vi "Deinitialize.vi"(8 "error in":errorcluster, 11 "Channel":u16) -> (0 "error out":errorcluster)   [LabVIEW 2023, in "PCAN API.lvlib"]
doc: "This VI is used to deinitialize a CAN port."
uses:
  PCAN API.lvlib
  PCAN2023/PCAN2023.lvlib
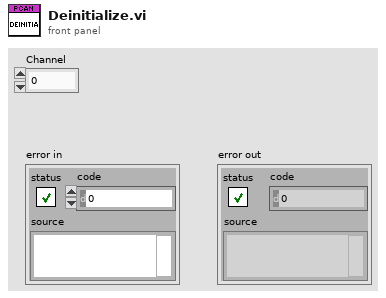
[diagram p1: front panel]
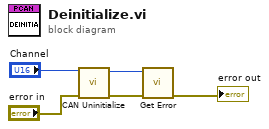
[diagram p0: block diagram]
diagram:
  n1 = call "CAN Uninitialize.vi"("error in (no error)"="error in", "Channel"="Channel") -> ("error out"=w3:errorcluster, "function return"=w1:u32)  [unwired: 8 in]
  n2 = call "Get Error.vi"("error in (no error)"=w3, "function return"=w1) -> ("error out"=→"error out":errorcluster)  [unwired: 9 in]
